vi "QuoteUnquotedString.vi"(10 "String in":string) -> (2 "String out":string)   [LabVIEW 2023]
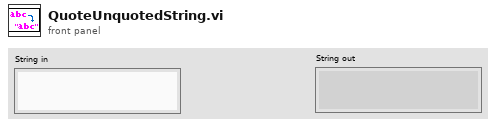
[diagram p1: front panel]
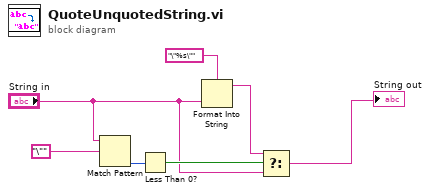
[diagram p0: block diagram]
diagram:
  n1 = Match Pattern(string="String in", regular expression="\"") -> (offset past match=w6:i32)  [unwired: 1 in, 3 out]
  n2 = Less Than 0?(x=w6) -> (x < 0?=w5:bool)
  n3 = Format Into String(format string="\"%s\"", "String in") -> (resulting string=w1:string)  [unwired: 2 in, 1 out]
  n4 = Select(t=w1, s=w5, f="String in") -> (s? t:f=→"String out":string)
